vi "Write Device Info.vi"(10 "device information":T1 {"capability_flags" format="%.0x"; "serial" format="%.0x"}, 11 "log file":path=path "c:/ni-rt/VeriStand/Custom Devices/AIM ARINC 429 debug log.txt") -> (0 "error out":errorcluster)   [LabVIEW 2020]
uses:
  <instrlib>/_AIM 429/Session/controls/api429_board_info.ctl
  <instrlib>/_AIM 429/Session/Session.lvclass
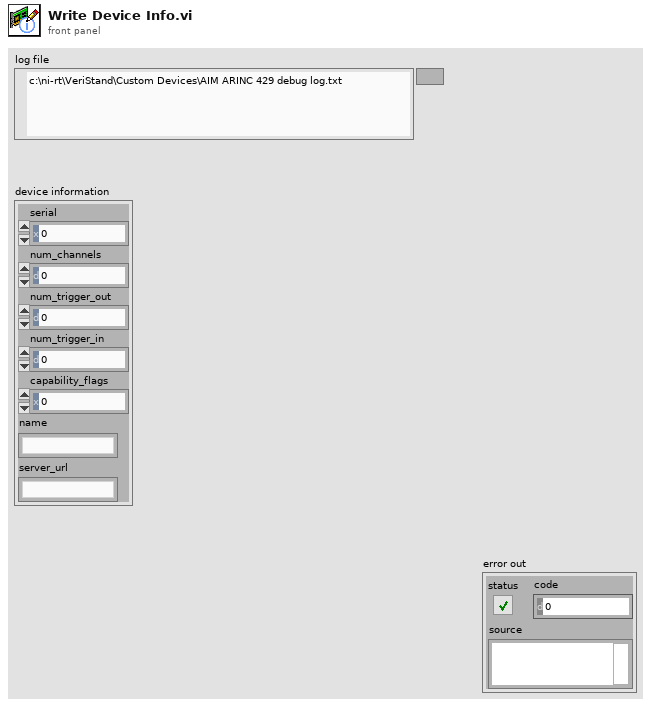
[diagram p1: front panel]
types:
  T1 = typedef "AIM429LV.lvlib/Session.lvclass/api429_board_info.ctl" = cluster{"serial":u32, "num_channels":u32, "num_trigger_out":u32, "num_trigger_in":u32, "capability_flags":u32, "name":string, "server_url":string}
  T2 = cluster{"serial":string, "num_channels":u32, "num_trigger_out":u32, "num_trigger_in":u32, "capability_flags":string, "name":string, "server_url":string}
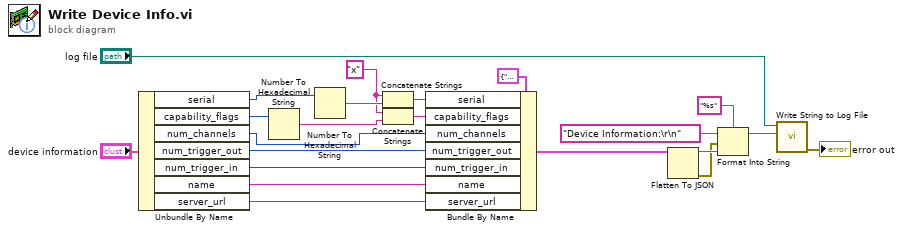
[diagram p0: block diagram]
diagram:
  w2 = "x" ("string")
  n1 = Unbundle By Name("device information") -> ("serial"=w13:u32, "capability_flags"=w12:u32, "num_channels"=w11:u32, "num_trigger_out"=w10:u32, "num_trigger_in"=w9:u32, "name"=w8:string, "server_url"=w7:string)
  n2 = Number To Hexadecimal String(2:w12) -> (0:w1:string)  [unwired: 1 in]
  n3 = Number To Hexadecimal String(2:w13) -> (0:w5:string)  [unwired: 1 in]
  n4 = Concatenate Strings(w2, w5) -> (w4:string)
  n5 = Concatenate Strings(w2, w1) -> (w3:string)
  n6 = Bundle By Name(cluster=T2 {"serial"="", "num_channels"=32, "num_trigger_out"=1, "num_trigger_in"=1, "capability_flags"="", "name"="Do you know?", "server_url"="www.ni.com"} ("device information"), "serial"=w4, "capability_flags"=w3, "num_channels"=w11, "num_trigger_out"=w10, "num_trigger_in"=w9, "name"=w8, "server_url"=w7) -> (w6:T2)
  n7 = Flatten To JSON(anything=w6) -> (JSON string=w22:string, 11:w21:errorcluster)  [unwired: 2 in]
  n8 = Format Into String(format string="%s", initial string="Device Information:\r\n", error in=w21, w22) -> (resulting string=w18:string)  [unwired: 1 out]
  n9 = call "Write String to Log File.vi"("string to log"=w18, "log file"="log file") -> ("error out"=→"error out":errorcluster)  [unwired: 9 in]
